vi "Setup.vi"(6 "HPF enable":bool, 7 "Queue Cluster":T1, 8 "error in (no error)":errorcluster, 10 "SR":u16=7812, 11 "LNAX301 in":refnum<class "LNAX301.lvclass">) -> (0 "error out":errorcluster, 3 "LNAX301 out":refnum<class "LNAX301.lvclass">)   [LabVIEW 2017, in "LNAX301.lvclass"]
uses:
  LNAX301.lvclass
  Ctl/MEMS.ctl
  ModbusRTUCmd.ctl
  Process/Process.ctl
  Caculator/Caculator.ctl
  LNAX301.lvclass/LNAX301.ctl
  DLL/Modbus.dll
panel:
  out "Chip ID":u16[](array[numeric])
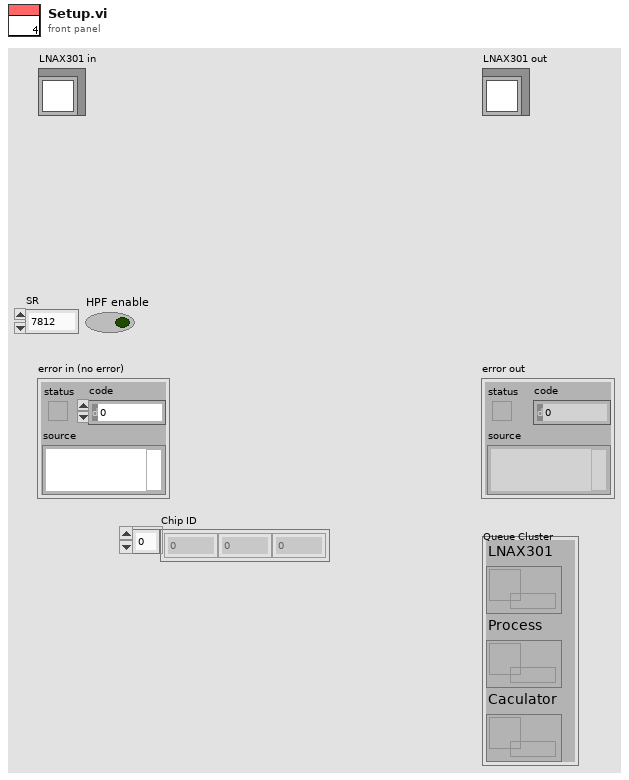
[diagram p1: front panel]
types:
  T1 = typedef "MEMS.ctl" = cluster{"LNAX301":refnum<queue>, "Process":refnum<queue>, "Caculator":refnum<queue>}
  T2 = typedef "Process.ctl" = cluster{"cmd":enum16{"Idle", "ini", "CheckData", "Disconnect", "UpdateSetup", "UpdateInstance", "Exit"}, "Var":variant}
  T3 = typedef "Caculator.ctl" = cluster{"cmd":enum16{"Idle", "ini", "Disconnect", "UpdateSetup", "ChangeView", "Caculator", "Exit"}, "Var":variant}
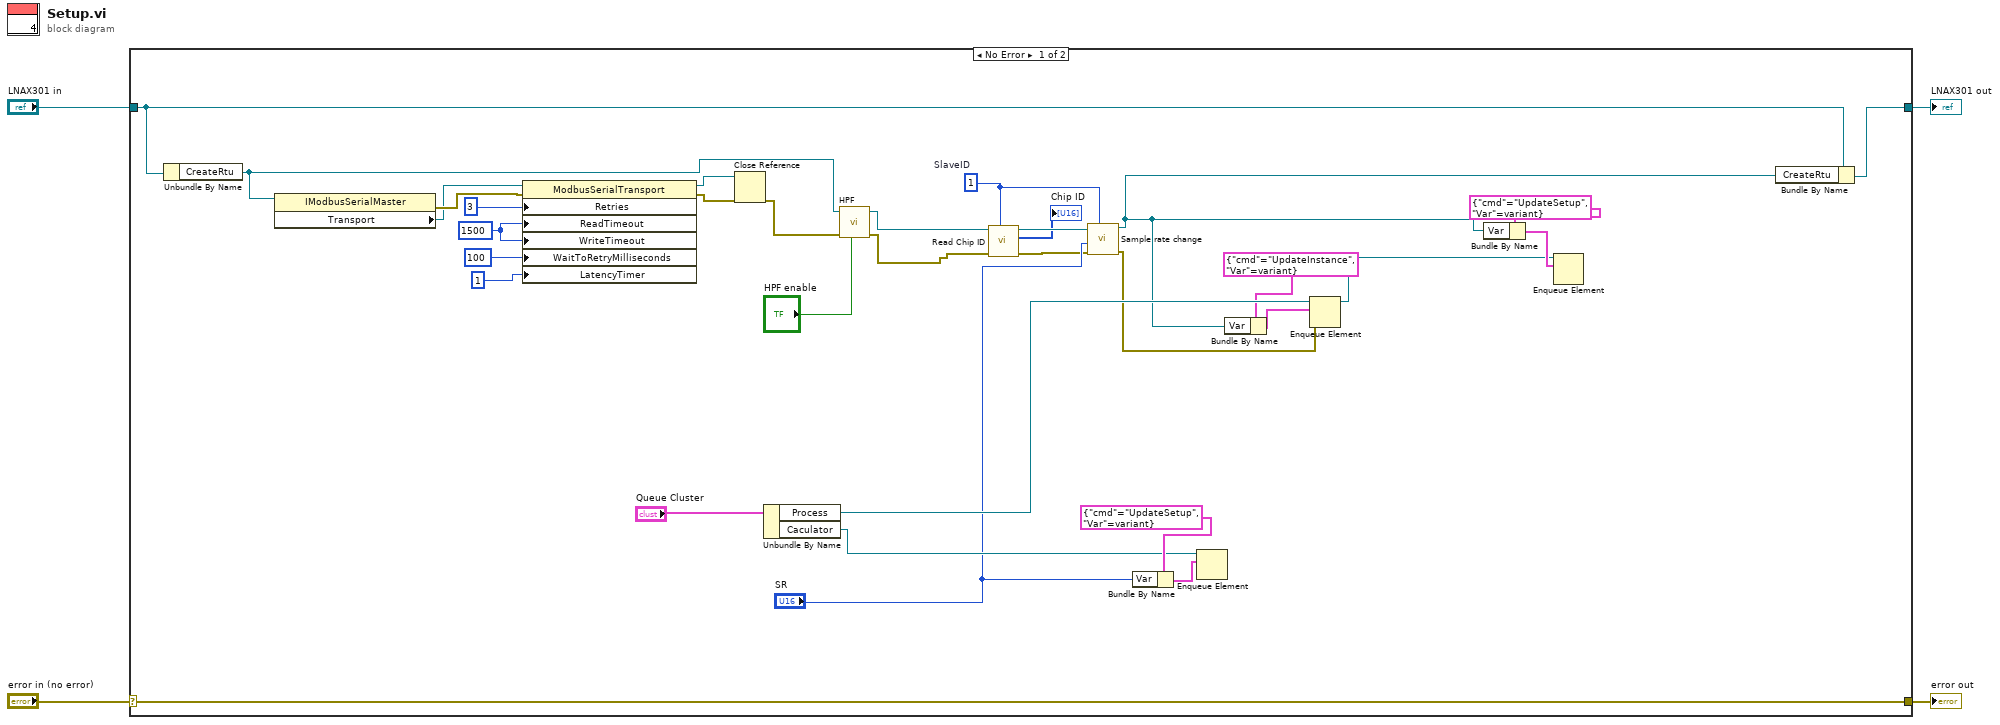
[diagram p0: block diagram]
diagram:
  n1 = case shown="No Error" "error in (no error)" {
    selector: "error in (no error)" -> [w37 w39]
    tunnel: [w37 w39] -> w3
    tunnel: [w35 w38] -> w1
    tunnel: "LNAX301 in" -> [w36 w38]
    frame No Error {
      w14 = u8 1  # SlaveID
      w20 = 1500 ("ReadTimeout")
      n2 = Unbundle By Name(w36) -> ("CreateRtu"=w9:refnum<k24>)
      n3 = property class="IModbusSerialMaster"(reference=w9) -> (error out=w23:errorcluster, "Transport"=w22:refnum<k24>)  [unwired: 1 in, 1 out]
      n4 = property class="ModbusSerialTransport"(reference=w22, error in=w23, "Retries"=3, "ReadTimeout"=w20, "WriteTimeout"=w20, "WaitToRetryMilliseconds"=100, "LatencyTimer"=1) -> (reference out=w24:refnum<k24>, error out=w25:errorcluster)
      n5 = Close Reference(reference=w24, error in (no error)=w25) -> (error out=w7:errorcluster)
      n6 = Unbundle By Name("Queue Cluster") -> ("Process"=w31:refnum<queue>, "Caculator"=w30:refnum<queue>)
      n7 = call "HPF.vi"("HPF enable"="HPF enable", "error in (no error)"=w7, "reference"=w9) -> ("error out"=w6:errorcluster, "reference out"=w8:refnum<k24>)  [unwired: 7 in]
      n8 = call "Read Chip ID.vi"("SlaveID"=w14, "error in (no error)"=w6, ".NET Refnum in"=w8) -> ("error out"=w17:errorcluster, "32bit integer"=→"Chip ID":i32[], ".NET Refnum out"=w16:refnum<k24>)  [unwired: 6 in]
      n9 = call "Sample rate change.vi"("SlaveID"=w14, "error in (no error)"=w17, "Sample Rate"="SR", ".NET Refnum in"=w16) -> ("error out"=w11:errorcluster, ".NET Refnum out"=w10:refnum<k24>)  [unwired: 6 in]
      n10 = Bundle By Name(cluster=T3 {"cmd"=enum."UpdateSetup", "Var"=variant} ("element"), "Var"="SR") -> (w33:T3)
      n11 = Enqueue Element(queue=w30, element=w33) -> ()  [unwired: 2 in, 3 out]
      n12 = Bundle By Name(cluster=T2 {"cmd"=enum."UpdateInstance", "Var"=variant} ("element"), "Var"=w10) -> (w13:T2)
      n13 = Enqueue Element(queue=w31, element=w13, error in (no error)=w11) -> (queue out=w27:refnum<queue>)  [unwired: 1 in, 2 out]
      n14 = Bundle By Name(cluster=T2 {"cmd"=enum."UpdateSetup", "Var"=variant} ("element"), "Var"=w10) -> (w29:T2)
      n15 = Enqueue Element(queue=w27, element=w29) -> ()  [unwired: 2 in, 3 out]
      n16 = Bundle By Name(cluster=w36, "CreateRtu"=w10) -> (w35:refnum<class "LNAX301.lvclass">)
    }
    frame Error {
    }
  }
  "error out" <- w3
  "LNAX301 out" <- w1
